vi "ZK_Findsolution.vi"(10 "Array":dbl[][](array[numeric])=[[0.0, 1.0, 0.0, 0.0, 0.0, 0.0, 0.0, 1.0], [0.0, 0.0, 0.0, 0.0, 0.0, 0.0, 0.0, 0.0], [0.0, 0.0, 0.0, 0.0, 0.0, 0.0, 1.0, 0.0], [0.0, 0.0, 0.0, 0.0, 0.0, 0.0, 0.0, 1.0], [0.0, 0.0, 0.0, 0.0, 0.0, 0.0, 0.0, 0.0], [0.0, 0.0, 1.0, 0.0, 0.0, 0.0, 1.0, 0.0], [0.0, 0.0, 0.0, 0.0, 0.0, 0.0, 0.0, 1.0], [0.0, 1.0, 1.0, 0.0, 0.0, 0.0, 0.0, 0.0]]) -> (1 "f":bool, 2 "Result":T1)   [LabVIEW 2018]
panel:
  out "A_1":bool
  out "output cluster":T1
  out "Array 5":dbl[](array[numeric])
  out "ROW":i32[](array[numeric])
  out "COL":i32[](array[numeric])
  out "A_4":bool
  out "A_3":bool
  out "ROw":i32[](array[numeric])
  out "cOL":i32[](array[numeric])
  out "Array 4":dbl[](array[numeric])
  out "A_2":bool
  out "Array 3":dbl[](array[numeric])
  out "RoW":i32
  out "Col":i32
  out "A_Row 2":i32
  out "A_Col 2":i32
  out "B_Row 2":i32
  out "B_Col 2":i32
  out "Array 2":bool[](array[boolean])
  out "B_Col":i32
  out "B_Row":i32
  out "A_Col":i32
  out "A_Row":i32
  out "Row":i32
  out "Column":i32
  out "Found":bool
  # "0"
  # "1"
  # "2"
  # "3"
  # "4"
  # "5"
  # "6"
  # "7"
  # "0"
  # "1"
  # "2"
  # "3"
  # "4"
  # "5"
  # "6"
  # "7"
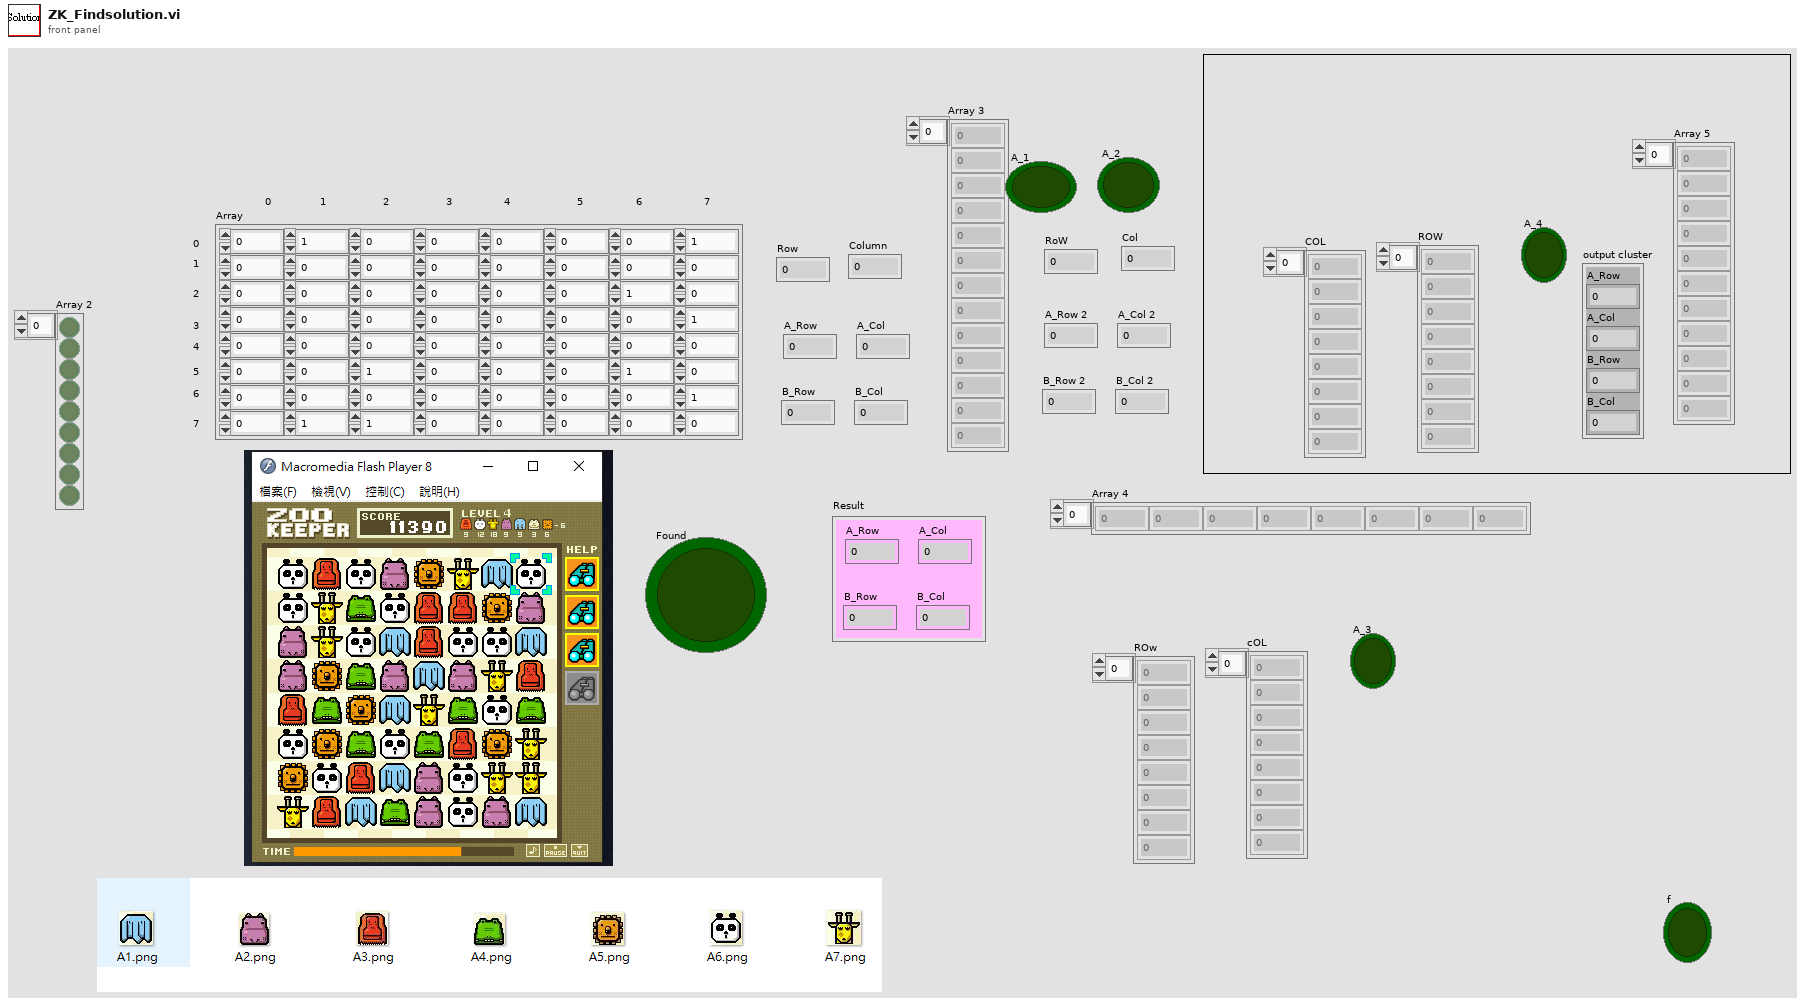
[diagram p1: front panel]
types:
  T1 = cluster{"A_Row":i32, "A_Col":i32, "B_Row":i32, "B_Col":i32}
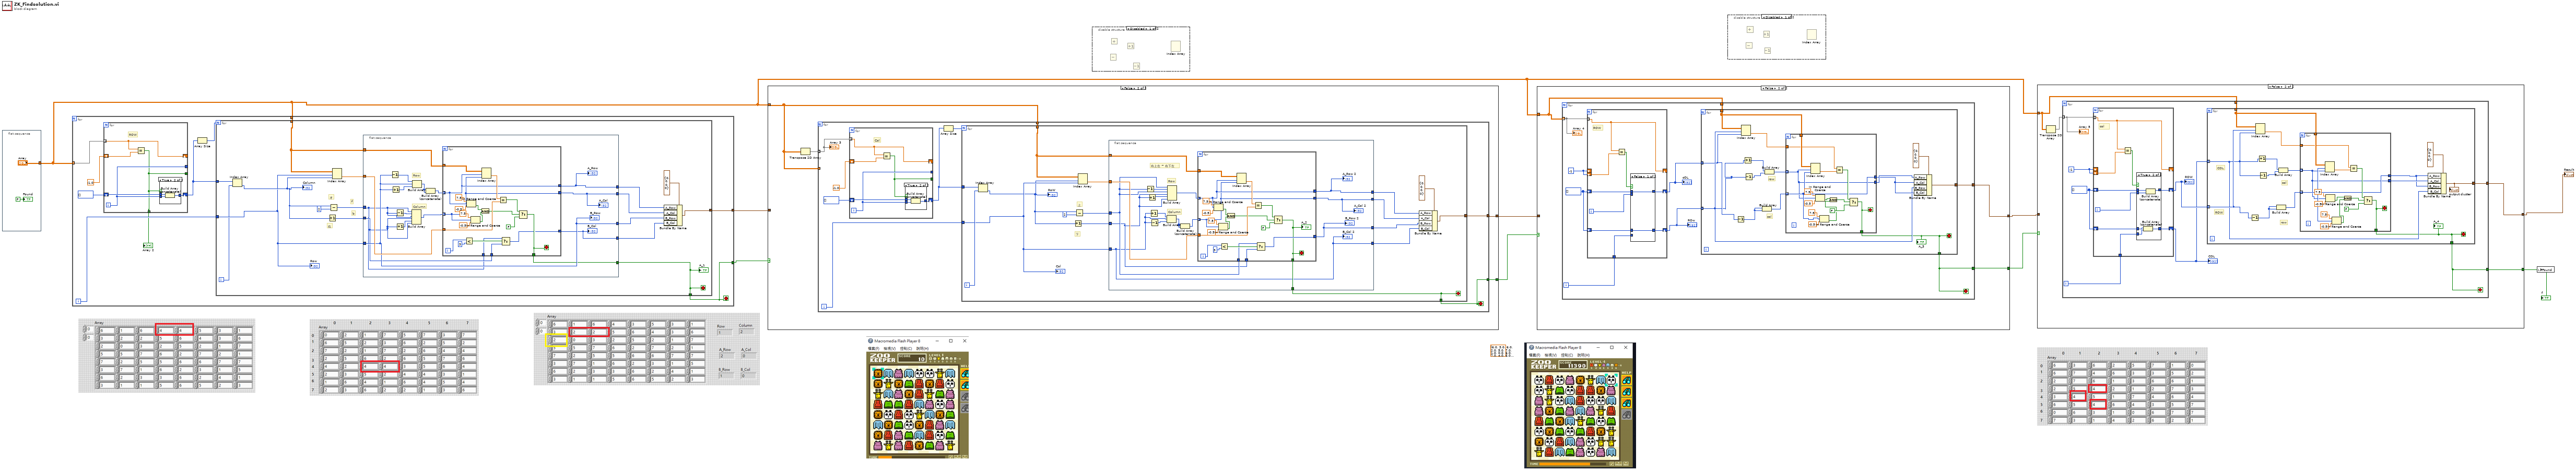
[diagram p0: block diagram]
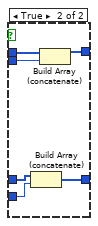
[diagram p6: hidden frame]
diagram:
  (unwired) dbl[][] [[6.0, 3.0, 6.0, 2.0, 5.0, 7.0, 1.0, 0.0], [6.0, 7.0, 4.0, 6.0, 3.0, 3.0, 5.0, 2.0], [2.0, 7.0, 6.0, 1.0, 3.0, 6.0, 6.0, 1.0], [2.0, 5.0, 4.0, 2.0, 1.0, 2.0, 7.0, 3.0], [3.0, 4.0, 5.0, 1.0, 7.0, 4.0, 6.0, 4.0], [6.0, 5.0, 4.0, 6.0, 4.0, 3.0, 5.0, 7.0], [0.0, 6.0, 3.0, 1.0, 0.0, 6.0, 7.0, 7.0], [7.0, 3.0, 1.0, 4.0, 2.0, 6.0, 2.0, 1.0]] ("Array")
  n1 = flat-sequence {
    tunnel: ["Array"] -> w4
    frame #0 {
      "Found" <- FALSE ("Found")
    }
  }
  n2 = for {
    tunnel: w4 -> [w21]
    tunnel: w4 -> [w18] mode=indexing
    tunnel: [w13] -> w8
    tunnel: [w12] -> w9
    i -> [w19]
    stop <- w12 stop-if-true
    n3 = for {
      tunnel: w18 -> [w79] mode=indexing
      shift-right: [w79] -> _
      shift-left: -1.0 -> [w80]
      tunnel: [w77] -> _
      tunnel: [w75] -> _
      tunnel: [w75] -> w16 mode=indexing
      shift-right: [w76] -> w15
      shift-left: i32[] [] -> [w78]
      i -> [w77]
      # "ROW"
      n4 = Equal?(x=w79, y=w80) -> (x = y?=w75:bool)
      n5 = case shown="True" w75 {
        tunnel: w78 -> [w81 w84]
        tunnel: w77 -> [_ w83]
        tunnel: [w81 w82] -> w76
        frame False {
        }
        frame True {
          n6 = Build Array (concatenate)(w84, w83) -> (w82:i32[])
        }
      }
    }
    "Array 2" <- w16
    n7 = Array Size(array=w15) -> (size(s)=w14:i32)
    n8 = for {
      N: w14 -> [_]
      tunnel: w21 -> [w37]
      tunnel: w19 -> [w33]
      tunnel: [w34] -> w12
      tunnel: w15 -> [w36]
      tunnel: [w31] -> w13
      i -> [w32]
      stop <- w34 stop-if-true
      # "右"
      # "オ"
      # "b"
      # "f"
      n9 = Index Array(array=w36, index=w32) -> (element=w35:i32)
      "Column" <- w35
      n10 = Increment(x=w35) -> (x+1=w27:i32)
      n11 = Subtract(x=w35, y=2) -> (x-y=w29:i32)
      n12 = Index Array(array=w37, index (row)=w33, index (col)=w35) -> (element=w28:dbl)
      n13 = flat-sequence {
        tunnel: w29 -> [w39]
        tunnel: w33 -> [w43]
        tunnel: w28 -> [w48]
        tunnel: w37 -> [w49]
        tunnel: w27 -> [w40]
        tunnel: [w44] -> w25
        tunnel: [w42] -> w24
        tunnel: [w43] -> w23
        tunnel: [w38] -> w22
        tunnel: [w41] -> w34
        frame #0 {
          # "Column"
          # "Row"
          n14 = Decrement(x=w43) -> (x-1=w53:i32)
          n15 = Increment(x=w43) -> (x+1=w51:i32)
          n16 = Decrement(x=w39) -> (x-1=w52:i32)
          n17 = Increment(x=w40) -> (x+1=w45:i32)
          n18 = Build Array(w39, w52, w39, w40, w45, w40) -> (w50:i32[])
          n19 = Build Array(w53, w43, w51) -> (w46:i32[])
          n20 = Build Array (concatenate)(w46, w46) -> (w47:i32[])
          n21 = for {
            tunnel: w47 -> [w59] mode=indexing
            tunnel: w50 -> [w55] mode=indexing
            tunnel: w49 -> [w74]
            tunnel: w48 -> [w72]
            tunnel: [w59] -> w44
            tunnel: [w55] -> w42
            tunnel: [w68] -> w41
            tunnel: w40 -> [w64]
            tunnel: w39 -> [w63]
            tunnel: [w62] -> w38
            i -> [w67]
            stop <- w68 stop-if-true
            n22 = Less?(x=w67, y=3) -> (x < y?=w65:bool)
            n23 = In Range and Coerce(upper limit=7.5, x=w59, lower limit=-0.5) -> (In Range?=w58:bool)  [unwired: 1 out]
            n24 = In Range and Coerce(upper limit=7.5, x=w55, lower limit=-0.5) -> (In Range?=w54:bool)  [unwired: 1 out]
            n25 = And(x=w58, y=w54) -> (x .and. y?=w71:bool)
            n26 = Index Array "Index Array"(array=w74, index (row)=w59, index (col)=w55) -> (element=w73:dbl)
            n27 = Equal?(x=w73, y=w72) -> (x = y?=w70:bool)
            n28 = Select(t=w63, s=w65, f=w64) -> (s? t:f=w62:i32)
            n29 = Select(t=w70, s=w71, f=FALSE) -> (s? t:f=w68:bool)
          }
          "A_Row" <- w44
          "A_Col" <- w42
          "B_Col" <- w38
          "B_Row" <- w43
        }
      }
      n30 = Bundle By Name(cluster=T1 {"A_Row"=0, "A_Col"=0, "B_Row"=0, "B_Col"=0} ("Cluster 2"), "A_Row"=w25, "A_Col"=w24, "B_Row"=w23, "B_Col"=w22) -> (w31:T1)
      "Row" <- w33
      "A_1" <- w34
    }
  }
  n31 = case shown="False" w9 {
    selector: w9 -> [w85 _]
    tunnel: w4 -> [_ w90]
    tunnel: [w86 w88] -> w6
    tunnel: w8 -> [w86 _]
    tunnel: [w85 w87] -> w7
    frame True {
    }
    frame False {
      n32 = Transpose 2D Array(2D array=w90) -> (transposed array=w89:dbl[][])
      n33 = for {
        tunnel: w90 -> [w99]
        tunnel: w90 -> [_] mode=indexing
        tunnel: [w93] -> w88
        tunnel: w89 -> [w92] mode=indexing
        tunnel: [w91] -> w87
        i -> [w97]
        stop <- w91 stop-if-true
        n34 = for {
          shift-right: [w153] -> _
          shift-left: -1.0 -> [w158]
          tunnel: [w156] -> _
          tunnel: [w154] -> _
          shift-right: [w155] -> w95
          shift-left: i32[] [] -> [w157]
          tunnel: w92 -> [w153] mode=indexing
          i -> [w156]
          # "Col"
          n35 = Equal?(x=w153, y=w158) -> (x = y?=w154:bool)
          n36 = case shown="True" w154 {
            tunnel: w157 -> [w159 w162]
            tunnel: w156 -> [_ w161]
            tunnel: [w159 w160] -> w155
            frame False {
            }
            frame True {
              n37 = Build Array (concatenate)(w162, w161) -> (w160:i32[])
            }
          }
        }
        n38 = Array Size(array=w95) -> (size(s)=w94:i32)
        n39 = for {
          N: w94 -> [_]
          tunnel: w99 -> [w115]
          tunnel: w97 -> [w102]
          tunnel: w95 -> [w114]
          tunnel: [w112] -> w93
          tunnel: [w103] -> w91
          i -> [w113]
          stop <- w103 stop-if-true
          # "上"
          # "下"
          n40 = Index Array(array=w114, index=w113) -> (element=w101:i32)
          "RoW" <- w101
          n41 = Increment(x=w101) -> (x+1=w108:i32)
          n42 = Subtract(x=w101, y=2) -> (x-y=w110:i32)
          n43 = Index Array(array=w115, index (row)=w101, index (col)=w102) -> (element=w109:dbl)
          n44 = flat-sequence {
            tunnel: w110 -> [w126]
            tunnel: w102 -> [w116]
            tunnel: w109 -> [w130]
            tunnel: w115 -> [w131]
            tunnel: w108 -> [w124]
            tunnel: [w118] -> w106
            tunnel: [w129] -> w105
            tunnel: [w116] -> w104
            tunnel: [w128] -> w103
            tunnel: [w117] -> w100
            frame #0 {
              # "右上左 ~ 右下左"
              # "Column"
              # "Row"
              n45 = Decrement(x=w126) -> (x-1=w127:i32)
              n46 = Increment(x=w124) -> (x+1=w125:i32)
              n47 = Increment(x=w116) -> (x+1=w123:i32)
              n48 = Decrement(x=w116) -> (x-1=w122:i32)
              n49 = Build Array(w123, w116, w122) -> (w120:i32[])
              n50 = Build Array(w126, w127, w126, w124, w125, w124) -> (w121:i32[])
              n51 = Build Array (concatenate)(w120, w120) -> (w119:i32[])
              n52 = for {
                tunnel: w121 -> [w137] mode=indexing
                tunnel: w119 -> [w133] mode=indexing
                tunnel: w131 -> [w152]
                tunnel: w130 -> [w150]
                tunnel: [w137] -> w118
                tunnel: [w133] -> w129
                tunnel: w124 -> [w143]
                tunnel: w126 -> [w142]
                tunnel: [w141] -> w117
                tunnel: [w140] -> w128
                i -> [w146]
                stop <- w140 stop-if-true
                n53 = In Range and Coerce(upper limit=7.5, x=w137, lower limit=-0.5) -> (In Range?=w136:bool)  [unwired: 1 out]
                n54 = In Range and Coerce(upper limit=7.5, x=w133, lower limit=-0.5) -> (In Range?=w132:bool)  [unwired: 1 out]
                n55 = Less?(x=w146, y=3) -> (x < y?=w144:bool)
                n56 = And(x=w136, y=w132) -> (x .and. y?=w149:bool)
                n57 = Index Array "Index Array"(array=w152, index (row)=w137, index (col)=w133) -> (element=w151:dbl)
                n58 = Equal?(x=w151, y=w150) -> (x = y?=w148:bool)
                n59 = Select(t=w142, s=w144, f=w143) -> (s? t:f=w141:i32)
                n60 = Select(t=w148, s=w149, f=FALSE) -> (s? t:f=w140:bool)
                "A_2" <- w140
              }
              "A_Row 2" <- w118
              "A_Col 2" <- w129
              "B_Row 2" <- w117
              "B_Col 2" <- w116
            }
          }
          n61 = Bundle By Name(cluster=T1 {"A_Row"=0, "A_Col"=0, "B_Row"=0, "B_Col"=0} ("Cluster 2"), "A_Row"=w106, "A_Col"=w105, "B_Row"=w100, "B_Col"=w104) -> (w112:T1)
          "Col" <- w102
        }
        "Array 3" <- w92
      }
    }
  }
  n62 = disable-structure shown="Disabled" {
    frame Disabled {
      n63 = Subtract() -> ()  [unwired: 2 in, 1 out]
      n64 = Add() -> ()  [unwired: 2 in, 1 out]
      n65 = Increment() -> ()  [unwired: 1 in, 1 out]
      n66 = Decrement() -> ()  [unwired: 1 in, 1 out]
      n67 = Index Array() -> ()  [unwired: 3 in, 1 out]
    }
    frame Enabled {
    }
  }
  n68 = case shown="False" w7 {
    selector: w7 -> [w163 _]
    tunnel: w4 -> [_ w167]
    tunnel: [w164 w166] -> w5
    tunnel: w6 -> [w164 _]
    tunnel: [w163 w165] -> w2
    frame True {
    }
    frame False {
      n69 = for {
        tunnel: w167 -> [w176] mode=indexing
        tunnel: w167 -> [w170]
        tunnel: [w169] -> w166
        tunnel: [w168] -> w165
        i -> [w173]
        stop <- w168 stop-if-true
        w174 = i32[] []
        w175 = -1
        n70 = for {
          tunnel: w176 -> [w213] mode=indexing
          shift-right: [w213] -> _
          shift-left: w175 -> [_]
          shift-left: w175 -> [w214]
          shift-right: [w210] -> w171
          shift-left: w174 -> [w212]
          shift-right: [w206] -> w172
          shift-left: w174 -> [w208]
          tunnel: w173 -> [w207]
          i -> [w211]
          # "ROW"
          n71 = Equal?(x=w213, y=w214) -> (x = y?=w209:bool)
          n72 = case shown="False" w209 {
            tunnel: w212 -> [w216 w222]
            tunnel: w211 -> [_ w221]
            tunnel: [w216 w220] -> w210
            tunnel: w208 -> [w215 w219]
            tunnel: w207 -> [_ w218]
            tunnel: [w215 w217] -> w206
            frame False {
            }
            frame True {
              n73 = Build Array (concatenate)(w219, w218) -> (w217:i32[])
              n74 = Build Array (concatenate)(w222, w221) -> (w220:i32[])
            }
          }
        }
        "cOL" <- w171
        "ROw" <- w172
        n75 = for {
          tunnel: w172 -> [w178] mode=indexing
          tunnel: w171 -> [w181] mode=indexing
          tunnel: w170 -> [w185]
          tunnel: [w183] -> w169
          tunnel: [w177] -> w168
          stop <- w177 stop-if-true
          # "col"
          # "row"
          n76 = Decrement(x=w181) -> (x-1=w179:i32)
          n77 = Index Array "Index Array"(array=w185, index (row)=w178, index (col)=w181) -> (element=w188:dbl)
          n78 = Increment(x=w178) -> (x+1=w190:i32)
          n79 = Decrement(x=w178) -> (x-1=w189:i32)
          n80 = Build Array(w179, w179) -> (w186:i32[])
          n81 = Build Array(w190, w189) -> (w187:i32[])
          n82 = for {
            tunnel: w188 -> [w204]
            tunnel: w187 -> [w192] mode=indexing
            tunnel: w186 -> [w196] mode=indexing
            tunnel: w185 -> [w205]
            tunnel: [w199] -> w177
            tunnel: [w196] -> w180
            tunnel: [w192] -> w182
            stop <- w199 stop-if-true
            n83 = Index Array "Index Array"(array=w205, index (row)=w192, index (col)=w196) -> (element=w203:dbl)
            n84 = In Range and Coerce(upper limit=7.5, x=w192, lower limit=-0.5) -> (In Range?=w191:bool)  [unwired: 1 out]
            n85 = In Range and Coerce(upper limit=7.5, x=w196, lower limit=-0.5) -> (In Range?=w195:bool)  [unwired: 1 out]
            n86 = And(x=w191, y=w195) -> (x .and. y?=w202:bool)
            n87 = Equal?(x=w204, y=w203) -> (x = y?=w200:bool)
            n88 = Select(t=w200, s=w202, f=FALSE) -> (s? t:f=w199:bool)
          }
          "A_3" <- w177
          n89 = Bundle By Name(cluster=T1 {"A_Row"=0, "A_Col"=0, "B_Row"=0, "B_Col"=0} ("Cluster 2"), "A_Row"=w182, "A_Col"=w180, "B_Row"=w178, "B_Col"=w180) -> (w183:T1)
        }
        "Array 4" <- w176
      }
    }
  }
  n90 = disable-structure shown="Disabled" {
    frame Disabled {
      n91 = Subtract() -> ()  [unwired: 2 in, 1 out]
      n92 = Add() -> ()  [unwired: 2 in, 1 out]
      n93 = Increment() -> ()  [unwired: 1 in, 1 out]
      n94 = Decrement() -> ()  [unwired: 1 in, 1 out]
      n95 = Index Array() -> ()  [unwired: 3 in, 1 out]
    }
    frame Enabled {
    }
  }
  n96 = case shown="False" w2 {
    selector: w2 -> [w223 _]
    tunnel: w4 -> [_ w227]
    tunnel: [w224 w228] -> w1
    tunnel: w5 -> [w224 _]
    tunnel: [w223 w225] -> w3
    frame True {
    }
    frame False {
      n97 = Transpose 2D Array(2D array=w227) -> (transposed array=w226:dbl[][])
      n98 = for {
        tunnel: w226 -> [w237] mode=indexing
        tunnel: w227 -> [w233]
        tunnel: [w232] -> w228
        tunnel: [w229] -> w225
        i -> [w234]
        stop <- w229 stop-if-true
        w235 = i32[] []
        w236 = -1
        n99 = for {
          tunnel: w237 -> [w274] mode=indexing
          shift-right: [w274] -> _
          shift-left: w236 -> [_]
          shift-left: w236 -> [w275]
          shift-right: [w271] -> w231
          shift-left: w235 -> [w273]
          shift-right: [w267] -> w230
          shift-left: w235 -> [w269]
          tunnel: w234 -> [w268]
          i -> [w272]
          # "col"
          n100 = Equal?(x=w274, y=w275) -> (x = y?=w270:bool)
          n101 = case shown="True" w270 {
            tunnel: w273 -> [w277 w283]
            tunnel: w272 -> [_ w282]
            tunnel: [w277 w281] -> w271
            tunnel: w269 -> [w276 w280]
            tunnel: w268 -> [_ w279]
            tunnel: [w276 w278] -> w267
            frame False {
            }
            frame True {
              n102 = Build Array (concatenate)(w280, w279) -> (w278:i32[])
              n103 = Build Array (concatenate)(w283, w282) -> (w281:i32[])
            }
          }
        }
        "ROW" <- w231
        "COL" <- w230
        n104 = for {
          tunnel: w231 -> [w242] mode=indexing
          tunnel: w230 -> [w239] mode=indexing
          tunnel: w233 -> [w246]
          tunnel: [w244] -> w232
          tunnel: [w238] -> w229
          stop <- w238 stop-if-true
          # "COL"
          # "ROW"
          # "col"
          # "row"
          n105 = Decrement(x=w242) -> (x-1=w243:i32)
          n106 = Index Array "Index Array"(array=w246, index (row)=w242, index (col)=w239) -> (element=w249:dbl)
          n107 = Increment(x=w239) -> (x+1=w251:i32)
          n108 = Decrement(x=w239) -> (x-1=w250:i32)
          n109 = Build Array(w243, w243) -> (w247:i32[])
          n110 = Build Array(w251, w250) -> (w248:i32[])
          n111 = for {
            tunnel: w249 -> [w265]
            tunnel: w248 -> [w253] mode=indexing
            tunnel: w247 -> [w257] mode=indexing
            tunnel: w246 -> [w266]
            tunnel: [w260] -> w238
            tunnel: [w257] -> w240
            tunnel: [w253] -> w241
            stop <- w260 stop-if-true
            n112 = Index Array "Index Array"(array=w266, index (row)=w257, index (col)=w253) -> (element=w264:dbl)
            n113 = In Range and Coerce(upper limit=7.5, x=w253, lower limit=-0.5) -> (In Range?=w252:bool)  [unwired: 1 out]
            n114 = In Range and Coerce(upper limit=7.5, x=w257, lower limit=-0.5) -> (In Range?=w256:bool)  [unwired: 1 out]
            n115 = And(x=w252, y=w256) -> (x .and. y?=w263:bool)
            n116 = Equal?(x=w265, y=w264) -> (x = y?=w261:bool)
            n117 = Select(t=w261, s=w263, f=FALSE) -> (s? t:f=w260:bool)
          }
          "A_4" <- w238
          n118 = Bundle By Name(cluster=T1 {"A_Row"=0, "A_Col"=0, "B_Row"=0, "B_Col"=0} ("Cluster 2"), "A_Row"=w240, "A_Col"=w241, "B_Row"=w240, "B_Col"=w239) -> (w244:T1)
          "output cluster" <- w244
        }
        "Array 5" <- w237
      }
    }
  }
  "Result" <- w1
  "f" <- w3
  n119 = local write "Found"(w3) -> ()
